vi "Do2.vi"(8 "error in (no error)":errorcluster, 10 "Numeric":dbl, 11 "Interface In":refnum<class>) -> (0 "error out":errorcluster, 2 "String":string, 3 "Interface Out":refnum<class>)   [LabVIEW 2016, in "Interface1.lvclass"]
uses:
  Interface1.lvclass
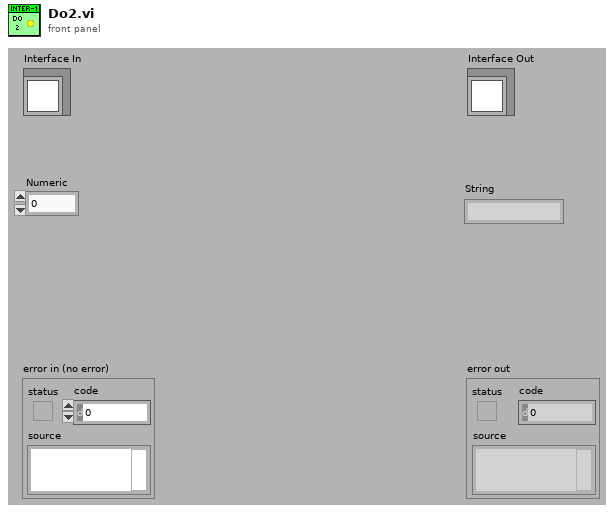
[diagram p1: front panel]
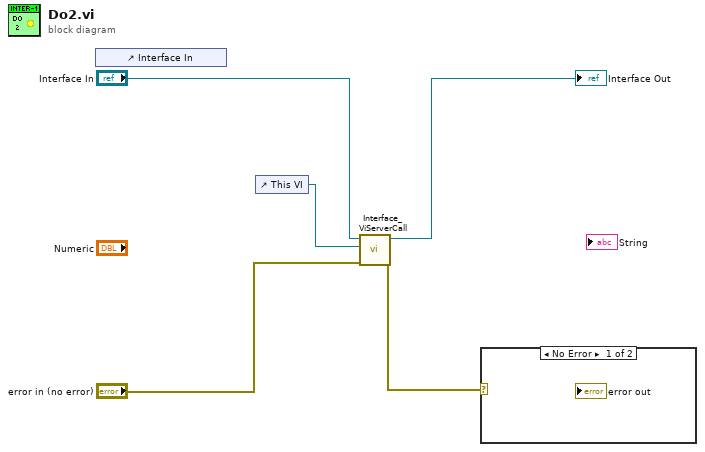
[diagram p0: block diagram]
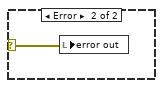
[diagram p2: hidden frame]
diagram:
  n1 = control-ref of="Interface In"() -> ()  [unwired: 1 out]
  n2 = control-ref of="This VI"() -> (w3:refnum<vi>)
  n3 = call <vilib>:"Interface_ViServerCall.vi"("error in (no error)"="error in (no error)", "Caller VI ref (This is the interface VI's reference)"=w3, "Interface In"="Interface In") -> ("error out"=w1:errorcluster, "Interface Out"=→"Interface Out":refnum<class>)  [unwired: 7 in]
  n4 = case shown="No Error" w1 {
    selector: w1 -> [_ w6]
    frame No Error {
    }
    frame Error {
      n5 = local write "error out"(w6) -> ()
    }
  }
